vi "getxy.vi"(4 "Fiber Num":i32, 6 "Error":bool, 7 "VISA resource name":refnum<visa-resource-name>="ASRL13::INSTR") -> (0 "y (CIE1931)":dbl, 1 "x (CIE1931)":dbl, 2 "Error":bool, 3 "dup VISA resource name":refnum<visa-resource-name>="ASRL13::INSTR")   [LabVIEW 2020, in "Library Instrument & Equipement.lvlib" / "Library LED Analyser.lvlib"]
uses:
  Library LED Analyser.lvlib
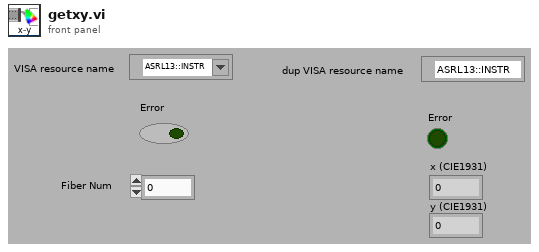
[diagram p1: front panel]
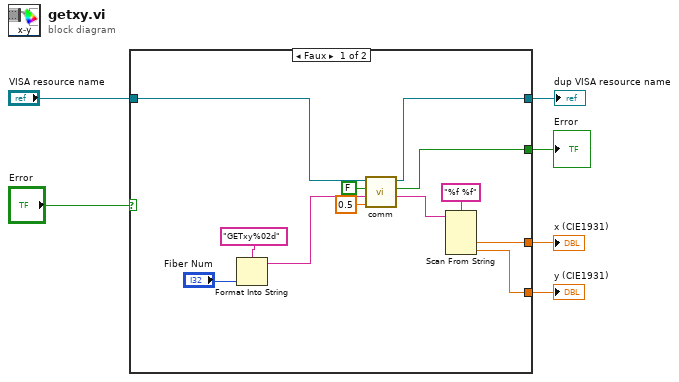
[diagram p0: block diagram]
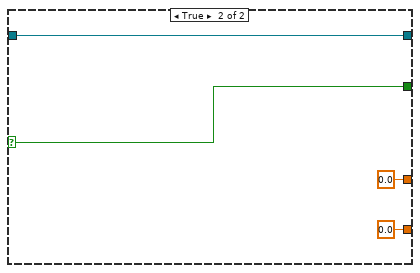
[diagram p2: hidden frame]
diagram:
  n1 = case shown="Faux" "Error" {
    selector: "Error" -> [_ w21]
    tunnel: "VISA resource name" -> [w18 w22]
    tunnel: [w11 0.0] -> w5
    tunnel: [w10 0.0] -> w4
    tunnel: [w8 w21] -> w2
    tunnel: [w7 w22] -> w1
    frame False {
      n2 = Format Into String(format string="GETxy%02d" ("Substring"), "Fiber Num") -> (resulting string=w15:string)  [unwired: 2 in, 1 out]
      n3 = call "comm.vi"("Timeout (s)"=0.5, "Command"=w15, "Error"=FALSE, "VISA resource name"=w18) -> ("Response"=w13:string, "Error"=w8:bool, "dup VISA resource name"=w7:refnum<visa-resource-name>)  [unwired: 2 in, 1 out]
      n4 = Scan From String(format string="%f %f", input string=w13) -> (output 1=w11:dbl, output 2=w10:dbl)  [unwired: 4 in, 3 out]
    }
    frame True {
    }
  }
  "x (CIE1931)" <- w5
  "y (CIE1931)" <- w4
  "Error" <- w2
  "dup VISA resource name" <- w1
